vi "Read Element of Array.vi"(10 "index":i32, 11 "CCD in":refnum<class "CCD.lvclass">) -> (2 "Image":T1, 3 "CCD out":refnum<class "CCD.lvclass">)   [LabVIEW 2016, in "Hardware.lvlib" / "CCD.lvlib" / "CCD.lvclass"]
uses:
  <userlib>/Common Components/Hardware/CCD/CCD/CCD.lvclass
  <vilib>/vision/Image Controls.llb/IMAQ Image.ctl
  <userlib>/Common Components/Hardware/CCD/CCD/CCD.lvclass/CCD.ctl
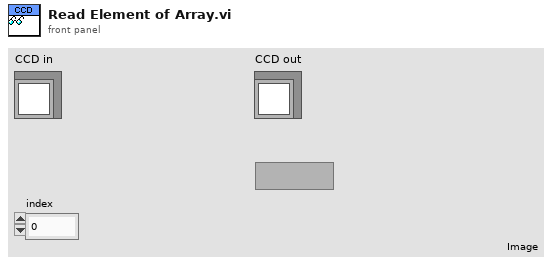
[diagram p1: front panel]
types:
  T1 = typedef "IMAQ Image.ctl" = refnum<image>
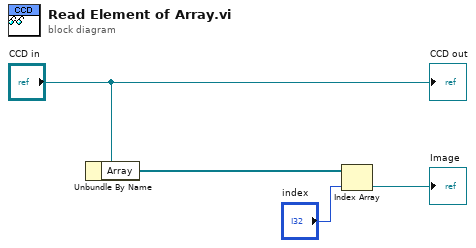
[diagram p0: block diagram]
diagram:
  n1 = Unbundle By Name("CCD in") -> ("Array"=w2:T1[])
  n2 = Index Array(array=w2, index="index") -> (element=→"Image":T1)
  "CCD out" <- "CCD in"
